vi "ConfigDevice.vi"(8 "error in (no error)":errorcluster, 11 "PacificPowerSource in":refnum<class "PacificPowerSource.lvclass">) -> (0 "error out":errorcluster, 3 "PacificPowerSource out":refnum<class "PacificPowerSource.lvclass">)   [LabVIEW 2018, in "AcPwrPlugins.lvlib" / "PacificPowerSource.lvclass"]
doc: "This VI configures the device based on the properties set in the preference dialog."
uses:
  PacificPowerSource.lvclass
  C:/Users/ico/Documents/Projects/NistPluggableModules/AcPwr/AcPwrPlugins/AcPwrBaseClass/AcPwrBase.lvclass
  AcPwrBaseClass/AcPwrBase.lvclass/AcPwrBase.ctl
  TypeDefs/ConfigDevicesModeSelection.ctl
  AcPwrBaseClass/Accessors/Read BaseConfig.vi
  <instrlib>/Pacific Power UPC Series/Pacific Power UPC Series.lvlib
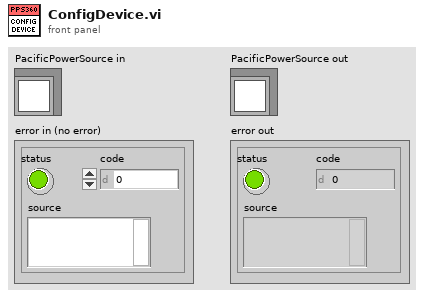
[diagram p1: front panel]
types:
  T1 = typedef "AcPwrPlugins.lvlib/PacificPowerSource.lvclass/ConfigDevicesModeSelection.ctl" = enum16{"Error", "ConfigureOutput", "VoltageLimit", "VoltageRange", "InitialVoltage", "FrequencyLimits", "FrequencyRange", "Impedance", "Waveform", "CustomWaveform", "Execute Program", "EnableOutput"}
  T2 = cluster{"Waveform 1":i32, "Waveform 2":i32, "Waveform 3":i32, "Voltage 1":dbl, "Voltage 2":dbl, "Voltage 3":dbl, "Phase 2":dbl, "Phase 3":dbl, "Frequency":dbl, "Current Limit":dbl, "# of Trans Events":i32, "Form":u16, "Coupling":u16, "XFMR Ratio":dbl, "Exec Angle":dbl}
  T3 = cluster{"Program Name":i32, "Waveform 1":i32, "Waveform 2":i32, "Waveform 3":i32, "Voltage 1":dbl, "Voltage 2":dbl, "Voltage 3":dbl, "Phase 2":dbl, "Phase 3":dbl, "Frequency":dbl, "Current Limit":dbl, "No. of Trans Events":i32, "Form":u16, "Coupling":u16, "XFMR Ratio":dbl, "Exec Angle":dbl}
  T4 = typedef "AcPwrPlugins.lvlib/AcPwrBase.lvclass/BaseConfig.ctl" = cluster{"Frequency":dbl, "FrequencyRange":dbl[], "Phases":T5[], "Name":string, "Chroma":T6, "NHRDC":T7, "PPS":T8, "PluginVariant":variant}
  T5 = typedef "AcPwrPlugins.lvlib/AcPwrBase.lvclass/Phase.ctl" = cluster{"Name":string, "Enabled":bool, "VoltageLevel":dbl, "Handle":string, "VoltageRange":dbl[], "Connected":bool, "CurrentLimit":dbl, "Waveform":string}
  T6 = typedef "AcPwrPlugins.lvlib/ChromaAcLoad.lvclass/DeviceProperties.ctl" = cluster{"Configuration Mode":enum16{"Constant Voltage (DC)", "Constant Power (DC)", "Constant Power (AC)", "Constant Current (DC)", "Constant Current (AC)", "Constant Resistance (DC)", "Constant Resistance (AC)", "Rectified Mode (DC)", "Inrush (AC)", "RLC CP (AC)", "RLC (AC)"}, "Phases":cluster{"Handle":string, "Name":string, "Phase Select":i32, "Instrument Options":string, "id query (T)":bool, "reset device (T)":bool, "Load Short Circuited":bool, "Line Synchronization":bool, "Load Current (A/Arms)":dbl, "Load Voltage (V/Vrms)":dbl, "Load Power (W)":dbl, "Load Resistance (Ohms)":dbl, "Load Current Peak Limit (A)":dbl, "Load Current Limit (A/Arms)":dbl, "Load Power Limit (W)":dbl, "Synch Frequency (Hz)":dbl, "Priority":enum16{"CF Only", "PF Only", "Both (CF)", "Both (PF)"}, "Crest Factor":dbl, "Power Factor":dbl, "Slew Rate":cluster{"Rise Slew Rate (A/ms)":i32, "Fall Slew Rate (A/ms)":i32}, "LC/RLC Mode":cluster{"Capacitance (uF)":i32, "Inductance (uH)":i32, "Series Resistance (Ohm)":dbl, "Parallel Resistance (Ohm)":dbl}, "Timing":cluster{"TimingOn":enum16{""}, "Hours":u32, "Minutes":u32, "Seconds":dbl, "CutoffVoltage":dbl}, "Connected":bool}[]}
  T7 = typedef "AcPwrPlugins.lvlib/NHRDCPower.lvclass/Device(s)Settings.ctl" = cluster{"Handle":string, "Name":string, "id query (Yes)":bool, "reset device (Yes)":bool, "Connected":bool, "Initial Battery Detect Voltage (0)":sgl, "SafetySettings":cluster{"SetWatchDog":bool, "Voltage (V)":sgl, "Current (A)":sgl, "Power (W)":sgl, "Voltage Delay (s)":sgl, "Current Delay (s)":sgl, "Power Delay (s)":sgl}, "Options String":string, "Aperture Time (s)":sgl, "operating state (Off)":i32, "OutputSettings":cluster{"Voltage (V)":sgl, "Current (A)":sgl, "Resistance (Ohms)":sgl, "Power (W)":sgl, "Enable Voltage":bool, "Enable Current":bool, "Enable Resistance":bool, "Enable Power":bool, "Delay After (s)":sgl, "Wait Value (V, A, W)":sgl, "Enable Wait":bool, "Wait on Value":i32}[], "SlewRate":cluster{"Set Voltage Rate V/S":dbl, "Set Current Rate A/S":dbl, "Set Resistance Rate R/S":dbl, "Set Power Rate W/S":dbl}}[]
  T8 = typedef "AcPwrPlugins.lvlib/PacificPowerSource.lvclass/DeviceSettings.ctl" = cluster{"Handle":string, "Connected":bool, "Clear Device (F)":bool, "btnIdQuery":bool, "btnReset":bool, "Program #":cluster{"Phase B (Degrees)":i32, "Waveform A (1: Sine)":i32, "Voltage Level (Va)":dbl, "Program Number (0)":i32, "Voltage Level (Vb) ":dbl, "Form (3: Three)":u16, "Coupling  (0: Direct)":u16, "Frequency (45Hz)":dbl, "Current Limit (40A)":dbl, "Phase C (Degrees)":i32, "Voltage Level (Vc)":dbl, "Waveform B (1: Sine)":i32, "Waveform C (1: Sine)":i32}[], "Impedance Parameters (off, 0.00)":cluster{"State":bool, "Impedance":dbl}, "Transient Execution (F)":bool, "OutputEnabled":bool, "Source Range":cluster{"Frequency Minimum (45 Hz)":dbl, "Frequency Maximum (1200 Hz)":dbl, "Voltage Maximum (V)":dbl, "Voltage Minimum (V)":dbl, "Range Control (0: Auto)":u16, "Initial Voltage (0V)":u16, "Frequency Range (600Hz)":u16}, "Port Type":enum16{"GPIB", "Serial"}}[]
  T9 = cluster{"Phase B (Degrees)":i32, "Waveform A (1: Sine)":i32, "Voltage Level (Va)":dbl, "Program Number (0)":i32, "Voltage Level (Vb) ":dbl, "Form (3: Three)":u16, "Coupling  (0: Direct)":u16, "Frequency (45Hz)":dbl, "Current Limit (40A)":dbl, "Phase C (Degrees)":i32, "Voltage Level (Vc)":dbl, "Waveform B (1: Sine)":i32, "Waveform C (1: Sine)":i32}[]
  T10 = cluster{"Phase B (Degrees)":i32, "Waveform A (1: Sine)":i32, "Voltage Level (Va)":dbl, "Program Number (0)":i32, "Voltage Level (Vb) ":dbl, "Form (3: Three)":u16, "Coupling  (0: Direct)":u16, "Frequency (45Hz)":dbl, "Current Limit (40A)":dbl, "Phase C (Degrees)":i32, "Voltage Level (Vc)":dbl, "Waveform B (1: Sine)":i32, "Waveform C (1: Sine)":i32}
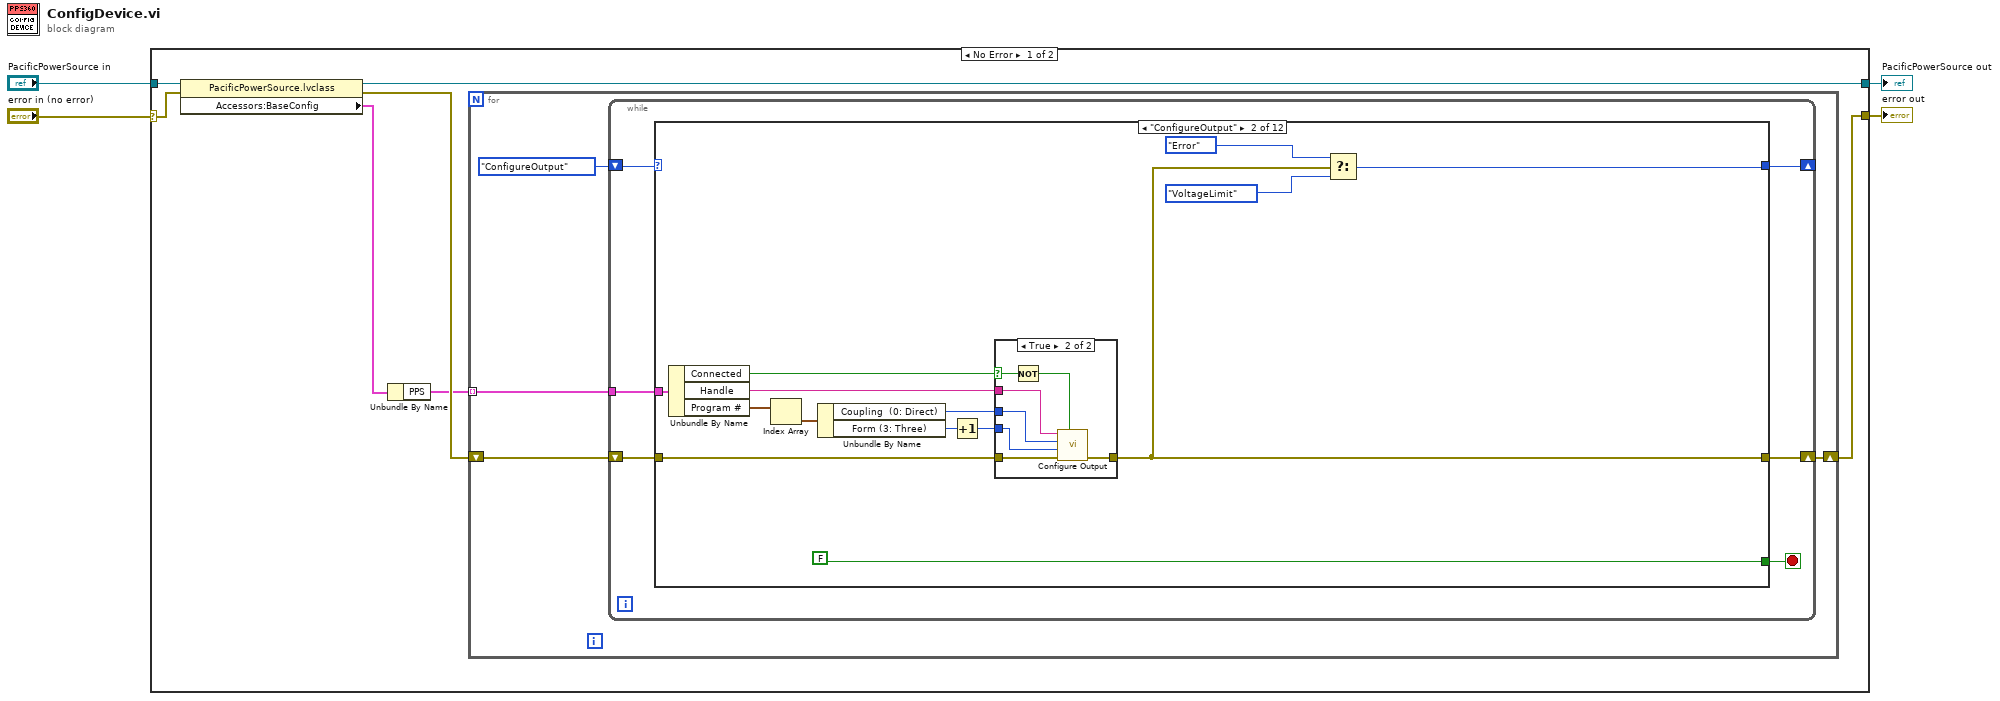
[diagram p0: block diagram]
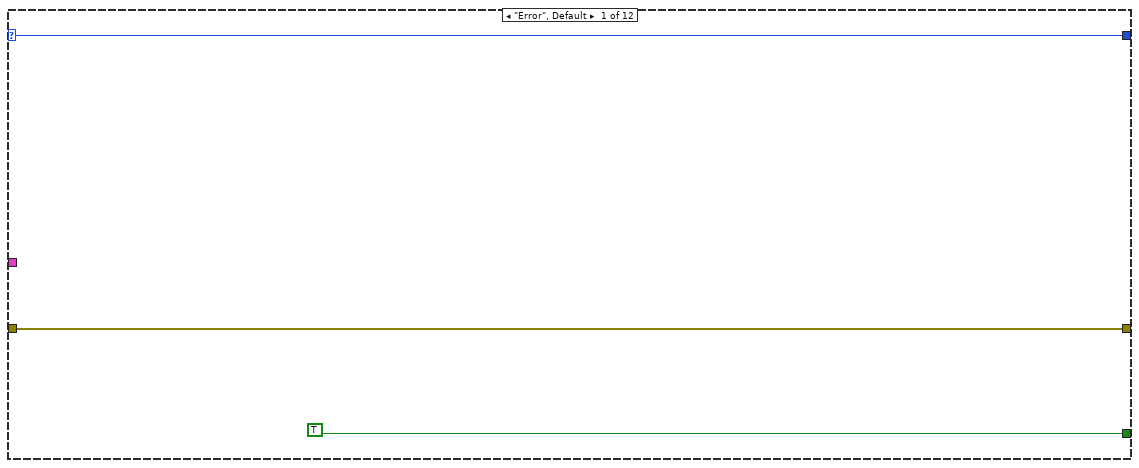
[diagram p2: hidden frame]
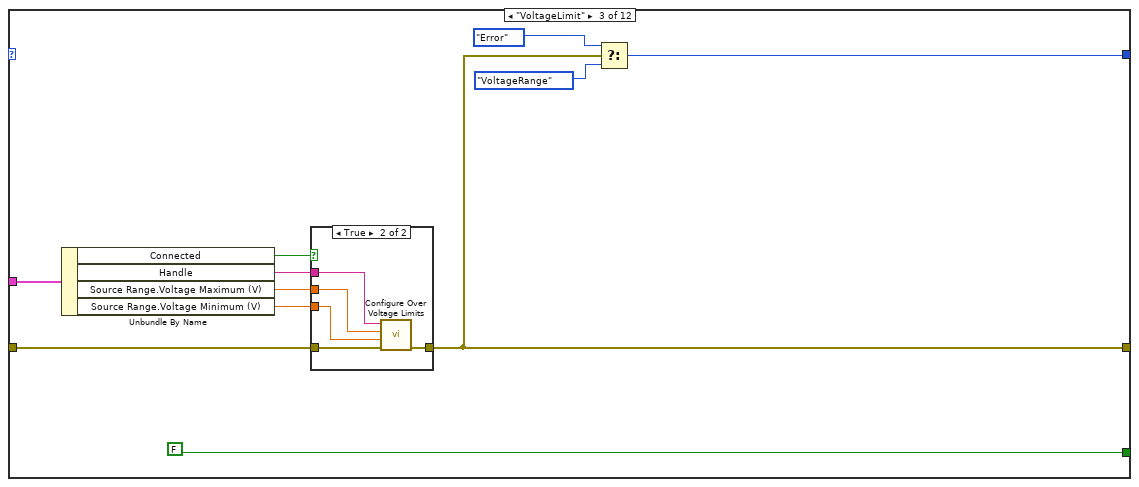
[diagram p4: hidden frame]
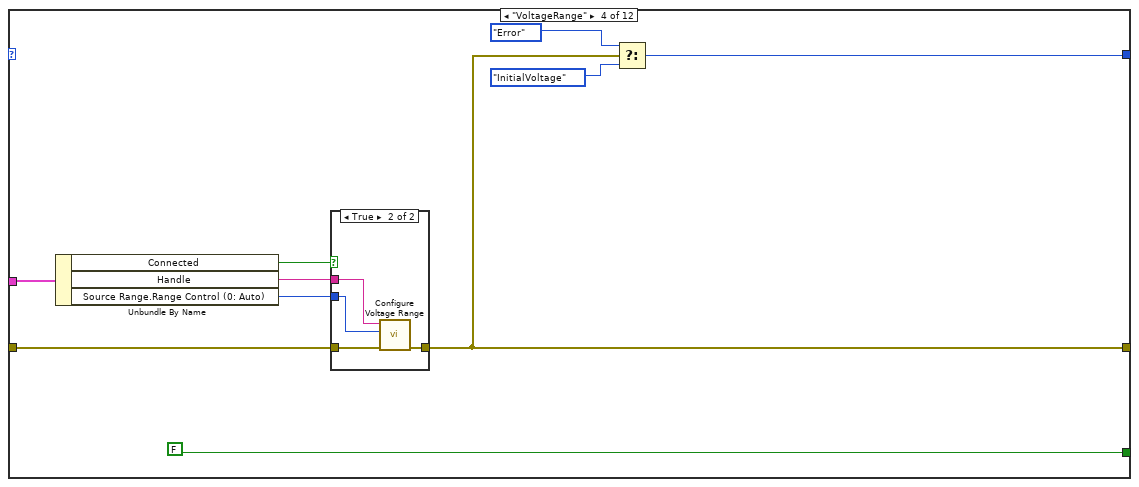
[diagram p6: hidden frame]
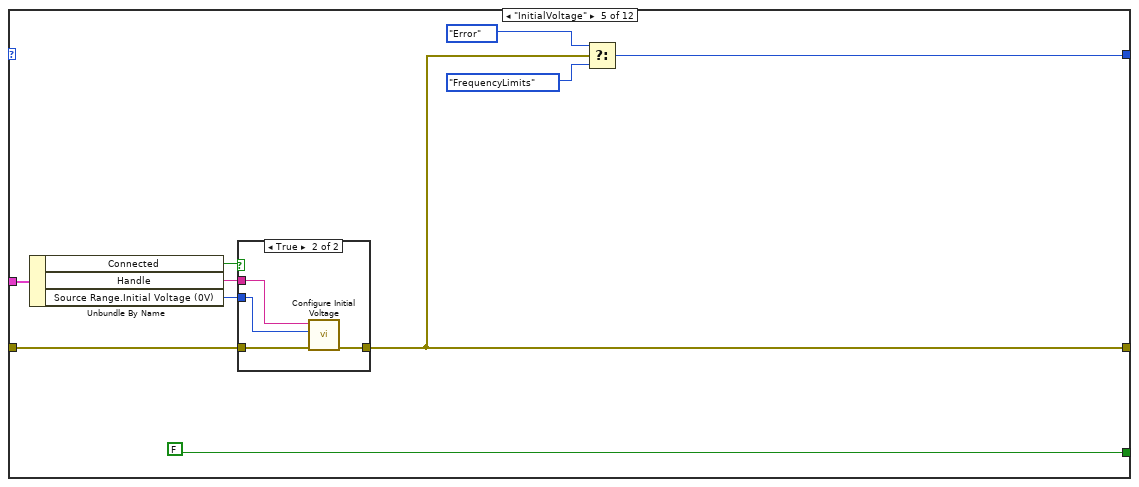
[diagram p8: hidden frame]
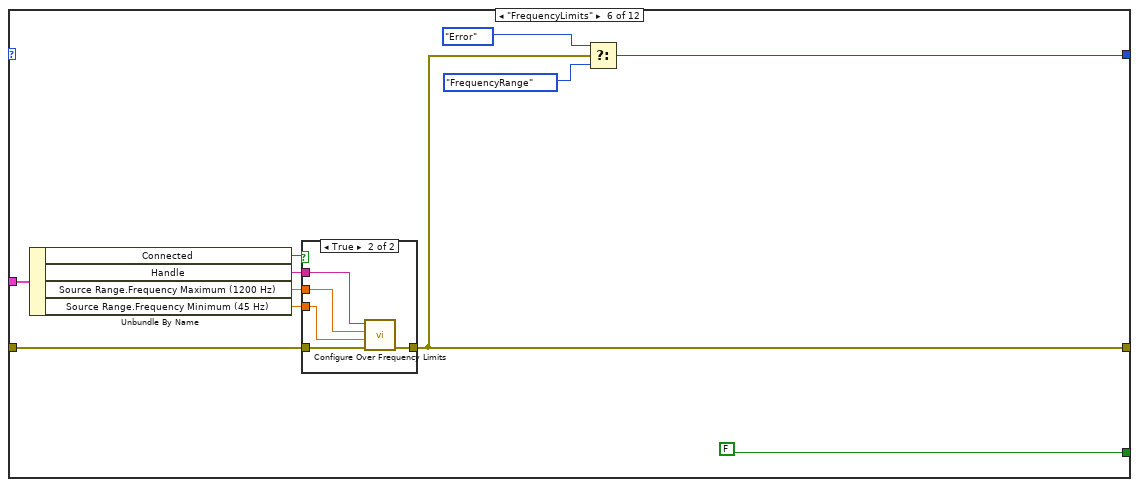
[diagram p10: hidden frame]
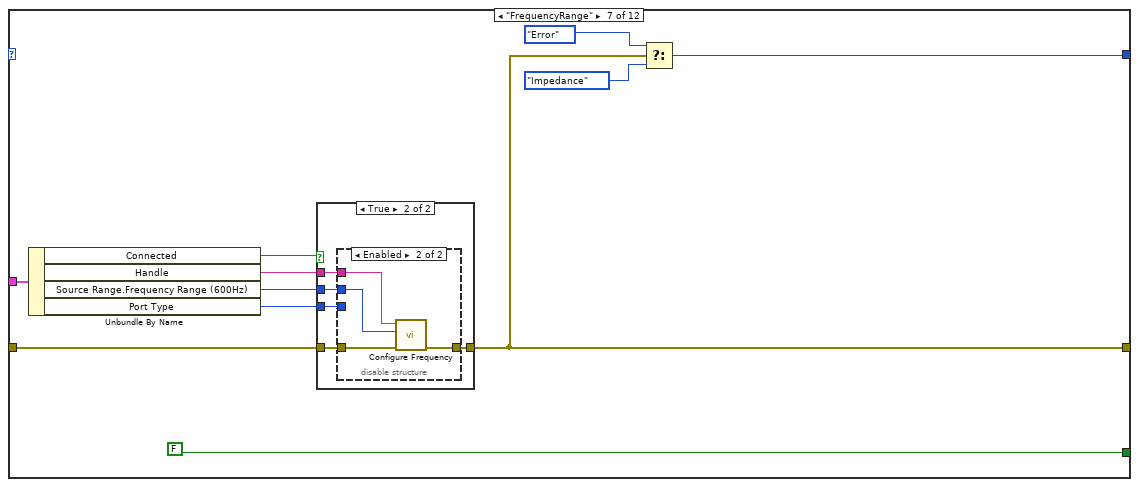
[diagram p12: hidden frame]
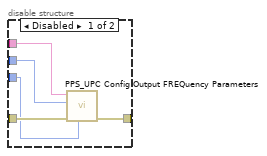
[diagram p14: hidden frame]
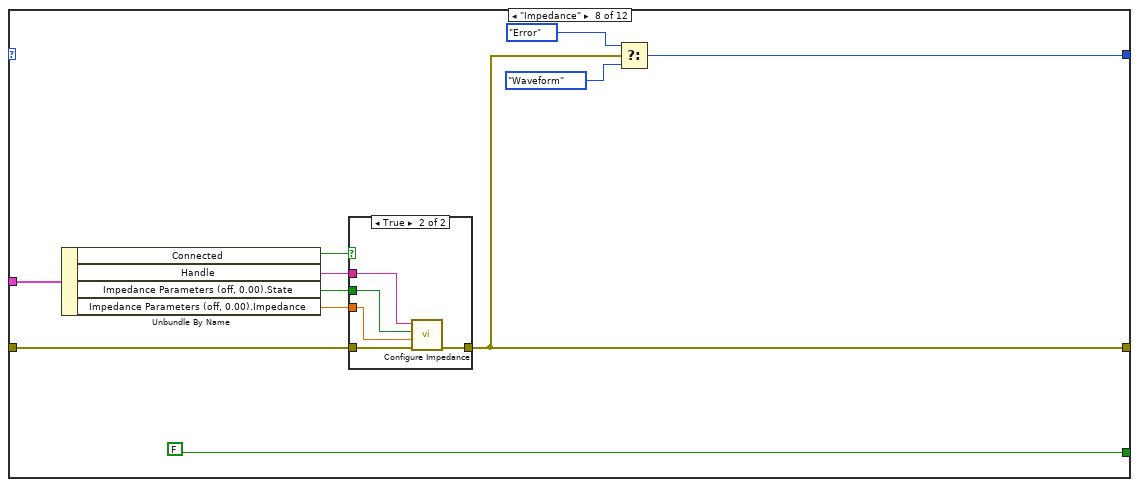
[diagram p15: hidden frame]
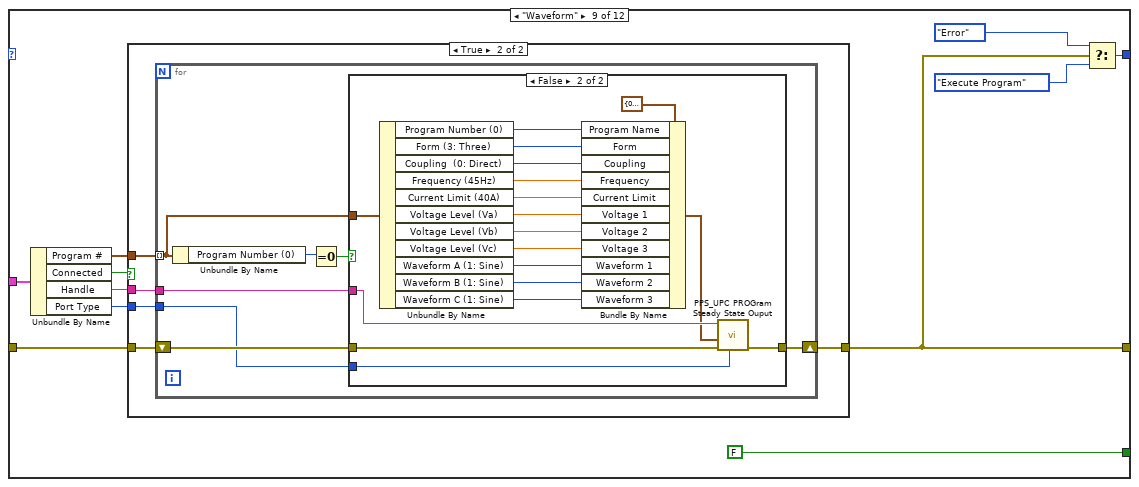
[diagram p17: hidden frame]
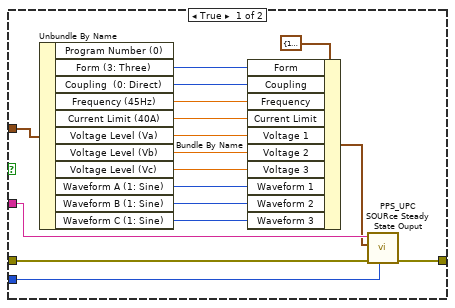
[diagram p19: hidden frame]
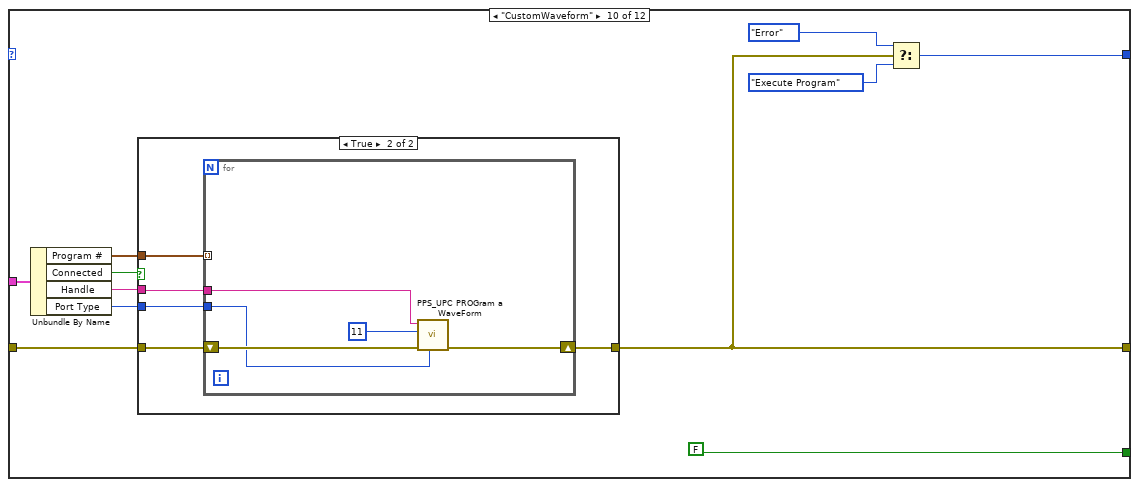
[diagram p20: hidden frame]
diagram:
  n1 = case shown="No Error" "error in (no error)" {
    selector: "error in (no error)" -> [w11 w278]
    tunnel: [w8 w278] -> w4
    tunnel: [w9 w277] -> w3
    tunnel: "PacificPowerSource in" -> [w10 w277]
    frame No Error {
      n2 = property class="PacificPowerSource.lvclass"(reference=w10, error in=w11) -> (reference out=w9:refnum<class "PacificPowerSource.lvclass">, error out=w7:errorcluster, "Accessors:BaseConfig"=w6:T4)
      n3 = Unbundle By Name(w6) -> ("PPS"=w5:T8)
      n4 = for {
        tunnel: w5 -> [w15] mode=indexing
        shift-right: [w13] -> w8
        shift-left: w7 -> [w14]
        n5 = while {
          tunnel: w15 -> [w21]
          shift-right: [w19] -> w13
          shift-left: w14 -> [w20]
          shift-right: [w16] -> _
          shift-left: ConfigDevicesModeSelection."ConfigureOutput" ("Enum") -> [w18]
          stop <- w17 stop-if-true
          n6 = case shown="\"ConfigureOutput\"" w18 {
            selector: w18 -> [w22 _ _ _ _ _ _ _ _ _ _ w259]
            tunnel: w21 -> [_ w32 w57 w73 w88 w104 w121 w140 w160 w219 w246 w264]
            tunnel: w20 -> [w24 w36 w54 w70 w84 w99 w117 w144 w162 w221 w247 w267]
            tunnel: [w24 w34 w52 w68 w82 w97 w115 w142 w155 w214 w244 w265] -> w19
            tunnel: [TRUE FALSE FALSE FALSE FALSE FALSE FALSE FALSE FALSE FALSE w235 TRUE] -> w17
            tunnel: [w22 w33 w51 w67 w81 w96 w114 w141 w156 w215 w242 w259] -> w16
            frame "Error", Default {
            }
            frame "ConfigureOutput" {
              n7 = Unbundle By Name(w32) -> ("Connected"=w38:bool, "Handle"=w37:string, "Program #"=w29:T9)
              n8 = Index Array(array=w29) -> (element=w28:T10)  [unwired: 1 in]
              n9 = Unbundle By Name(w28) -> ("Coupling  (0: Direct)"=w27:u16, "Form (3: Three)"=w26:u16)
              n10 = Increment(x=w26) -> (x+1=w25:u16)
              n11 = case shown="True" w38 {
                selector: w38 -> [_ w42]
                tunnel: w37 -> [_ w44]
                tunnel: w36 -> [w39 w45]
                tunnel: [w39 w46] -> w34
                tunnel: w27 -> [_ w43]
                tunnel: w25 -> [_ w40]
                frame False {
                }
                frame True {
                  n12 = Not(x=w42) -> (.not. x?=w41:bool)
                  n13 = call <instrlib>:"Configure Output.vi"("Enable Output (T: Enable)"=w41, "error in (no error)"=w45, "Form (3: Three)"=w40, "Coupling  (0: Direct)"=w43, "VISA resource name"=w44) -> ("error out"=w46:errorcluster)  [unwired: 5 in, 1 out]
                }
              }
              n14 = Select(t=ConfigDevicesModeSelection."Error" ("Enum"), s=w34, f=ConfigDevicesModeSelection."VoltageLimit" ("Enum")) -> (s? t:f=w33:T1)
            }
            frame "VoltageLimit" {
              n15 = Unbundle By Name(w57) -> ("Connected"=w50:bool, "Handle"=w56:string, "Source Range.Voltage Maximum (V)"=w55:dbl, "Source Range.Voltage Minimum (V)"=w49:dbl)
              n16 = case shown="True" w50 {
                tunnel: w56 -> [_ w61]
                tunnel: w55 -> [_ w60]
                tunnel: w54 -> [w58 w63]
                tunnel: [w58 w62] -> w52
                tunnel: w49 -> [_ w59]
                frame False {
                }
                frame True {
                  n17 = call <instrlib>:"Configure Over Voltage Limits.vi"("error in (no error)"=w63, "Low Limit (0.0 V)"=w59, "High Limit (600.0 V)"=w60, "VISA resource name"=w61) -> ("error out"=w62:errorcluster)  [unwired: 6 in, 1 out]
                }
              }
              n18 = Select(t=ConfigDevicesModeSelection."Error" ("Enum"), s=w52, f=ConfigDevicesModeSelection."VoltageRange" ("Enum")) -> (s? t:f=w51:T1)
            }
            frame "VoltageRange" {
              n19 = Unbundle By Name(w73) -> ("Connected"=w66:bool, "Handle"=w72:string, "Source Range.Range Control (0: Auto)"=w71:u16)
              n20 = case shown="True" w66 {
                tunnel: w72 -> [_ w76]
                tunnel: w71 -> [_ w75]
                tunnel: w70 -> [w74 w78]
                tunnel: [w74 w77] -> w68
                frame False {
                }
                frame True {
                  n21 = call <instrlib>:"Configure Voltage Range.vi"("error in (no error)"=w78, "Range Control (0: Auto)"=w75, "VISA resource name"=w76) -> ("error out"=w77:errorcluster)  [unwired: 7 in, 1 out]
                }
              }
              n22 = Select(t=ConfigDevicesModeSelection."Error" ("Enum"), s=w68, f=ConfigDevicesModeSelection."InitialVoltage" ("Enum")) -> (s? t:f=w67:T1)
            }
            frame "InitialVoltage" {
              n23 = Unbundle By Name(w88) -> ("Connected"=w87:bool, "Handle"=w86:string, "Source Range.Initial Voltage (0V)"=w85:u16)
              n24 = case shown="True" w87 {
                tunnel: w86 -> [_ w91]
                tunnel: w85 -> [_ w90]
                tunnel: w84 -> [w89 w92]
                tunnel: [w89 w93] -> w82
                frame False {
                }
                frame True {
                  n25 = call <instrlib>:"Configure Initial Voltage.vi"("error in (no error)"=w92, "Initial Voltage (0: 0 V)"=w90, "VISA resource name"=w91) -> ("error out"=w93:errorcluster)  [unwired: 7 in, 1 out]
                }
              }
              n26 = Select(t=ConfigDevicesModeSelection."Error" ("Enum"), s=w82, f=ConfigDevicesModeSelection."FrequencyLimits" ("Enum")) -> (s? t:f=w81:T1)
            }
            frame "FrequencyLimits" {
              n27 = Unbundle By Name(w104) -> ("Connected"=w103:bool, "Handle"=w102:string, "Source Range.Frequency Maximum (1200 Hz)"=w101:dbl, "Source Range.Frequency Minimum (45 Hz)"=w100:dbl)
              n28 = case shown="True" w103 {
                tunnel: w102 -> [_ w108]
                tunnel: w101 -> [_ w107]
                tunnel: w100 -> [_ w106]
                tunnel: w99 -> [w105 w109]
                tunnel: [w105 w110] -> w97
                frame False {
                }
                frame True {
                  n29 = call <instrlib>:"Configure Over Frequency Limits.vi"("error in (no error)"=w109, "Low Limit (45.0 Hz)"=w106, "High Limit (1200.0 Hz)"=w107, "VISA resource name"=w108) -> ("error out"=w110:errorcluster)  [unwired: 6 in, 1 out]
                }
              }
              n30 = Select(t=ConfigDevicesModeSelection."Error" ("Enum"), s=w97, f=ConfigDevicesModeSelection."FrequencyRange" ("Enum")) -> (s? t:f=w96:T1)
            }
            frame "FrequencyRange" {
              n31 = Unbundle By Name(w121) -> ("Connected"=w120:bool, "Handle"=w119:string, "Source Range.Frequency Range (600Hz)"=w118:u16, "Port Type"=w111:enum16{"GPIB", "Serial"})
              n32 = case shown="True" w120 {
                tunnel: w119 -> [_ w123]
                tunnel: w118 -> [_ w125]
                tunnel: w117 -> [w122 w126]
                tunnel: [w122 w127] -> w115
                tunnel: w111 -> [_ w124]
                frame False {
                }
                frame True {
                  n33 = disable-structure shown="Enabled" {
                    disable-tunnel: [w132 w135] -> w127
                    disable-tunnel: w126 -> [w131 w136]
                    disable-tunnel: w125 -> [w130 w133]
                    disable-tunnel: w124 -> [w129 _]
                    disable-tunnel: w123 -> [w128 w134]
                    frame Disabled {
                      n34 = call <instrlib>:"PPS_UPC Config Output FREQuency Parameters.vi"("Port Type"=w129, "error in (no error)"=w131, "Frequency Span (600)"=w130, "VISA session"=w128) -> ("error out"=w132:errorcluster)  [unwired: 6 in, 1 out]
                    }
                    frame Enabled {
                      n35 = call <instrlib>:"Configure Frequency.vi"("error in (no error)"=w136, "Frequency Range (600 Hz)"=w133, "VISA resource name"=w134) -> ("error out"=w135:errorcluster)  [unwired: 7 in, 1 out]
                    }
                  }
                }
              }
              n36 = Select(t=ConfigDevicesModeSelection."Error" ("Enum"), s=w115, f=ConfigDevicesModeSelection."Impedance" ("Enum")) -> (s? t:f=w114:T1)
            }
            frame "Impedance" {
              n37 = Unbundle By Name(w140) -> ("Connected"=w147:bool, "Handle"=w146:string, "Impedance Parameters (off, 0.00).State"=w145:bool, "Impedance Parameters (off, 0.00).Impedance"=w139:dbl)
              n38 = case shown="True" w147 {
                tunnel: w146 -> [_ w151]
                tunnel: w145 -> [_ w150]
                tunnel: w144 -> [w148 w152]
                tunnel: [w148 w153] -> w142
                tunnel: w139 -> [_ w149]
                frame False {
                }
                frame True {
                  n39 = call <instrlib>:"Configure Impedance.vi"("error in (no error)"=w152, "Output Impedance (0.0 Ohm)"=w149, "Enable Impedance (T: Enable)"=w150, "VISA resource name"=w151) -> ("error out"=w153:errorcluster)  [unwired: 6 in, 1 out]
                }
              }
              n40 = Select(t=ConfigDevicesModeSelection."Error" ("Enum"), s=w142, f=ConfigDevicesModeSelection."Waveform" ("Enum")) -> (s? t:f=w141:T1)
            }
            frame "Waveform" {
              n41 = Unbundle By Name(w160) -> ("Program #"=w159:T9, "Connected"=w164:bool, "Handle"=w163:string, "Port Type"=w154:enum16{"GPIB", "Serial"})
              n42 = case shown="True" w164 {
                tunnel: w163 -> [_ w168]
                tunnel: w162 -> [w165 w169]
                tunnel: [w165 w170] -> w155
                tunnel: w159 -> [_ w167]
                tunnel: w154 -> [_ w166]
                frame False {
                }
                frame True {
                  n43 = for {
                    shift-right: [w176] -> w170
                    shift-left: w169 -> [w177]
                    tunnel: w168 -> [w173]
                    tunnel: w167 -> [w172] mode=indexing
                    tunnel: w166 -> [w171]
                    n44 = Unbundle By Name(w172) -> ("Program Number (0)"=w175:i32)
                    n45 = Equal To 0?(x=w175) -> (x = 0?=w174:bool)
                    n46 = case shown="False" w174 {
                      tunnel: w177 -> [w194 w212]
                      tunnel: [w193 w201] -> w176
                      tunnel: w171 -> [w192 w200]
                      tunnel: w173 -> [w191 w199]
                      tunnel: w172 -> [w189 w211]
                      frame True {
                        n47 = Unbundle By Name(w189) -> ("Form (3: Three)"=w179:u16, "Coupling  (0: Direct)"=w180:u16, "Frequency (45Hz)"=w184:dbl, "Current Limit (40A)"=w185:dbl, "Voltage Level (Va)"=w188:dbl, "Voltage Level (Vb)"=w187:dbl, "Voltage Level (Vc)"=w186:dbl, "Waveform A (1: Sine)"=w183:i32, "Waveform B (1: Sine)"=w182:i32, "Waveform C (1: Sine)"=w181:i32)  [unwired: 1 out]
                        n48 = Bundle By Name(cluster=T2 {"Waveform 1"=1, "Waveform 2"=1, "Waveform 3"=1, "Voltage 1"=100.0, "Voltage 2"=100.0, "Voltage 3"=100.0, "Phase 2"=120.0, "Phase 3"=240.0, "Frequency"=100.0, "Current Limit"=10.0, "# of Trans Events"=0, "Form"=0, "Coupling"=0, "XFMR Ratio"=0.0, "Exec Angle"=0.0} ("Steady State Output Parameters 2"), "Form"=w179, "Coupling"=w180, "Frequency"=w184, "Current Limit"=w185, "Voltage 1"=w188, "Voltage 2"=w187, "Voltage 3"=w186, "Waveform 1"=w183, "Waveform 2"=w182, "Waveform 3"=w181) -> (w190:T2)
                        n49 = call <instrlib>:"PPS_UPC SOURce Steady State Ouput.vi"("Port Type"=w192, "error in (no error)"=w194, "Steady State\nOutput Parameters"=w190, "VISA session"=w191) -> ("error out"=w193:errorcluster)  [unwired: 6 in, 1 out]
                      }
                      frame False {
                        n50 = Unbundle By Name(w211) -> ("Program Number (0)"=w197:i32, "Form (3: Three)"=w198:u16, "Coupling  (0: Direct)"=w202:u16, "Frequency (45Hz)"=w206:dbl, "Current Limit (40A)"=w207:dbl, "Voltage Level (Va)"=w210:dbl, "Voltage Level (Vb)"=w209:dbl, "Voltage Level (Vc)"=w208:dbl, "Waveform A (1: Sine)"=w205:i32, "Waveform B (1: Sine)"=w204:i32, "Waveform C (1: Sine)"=w203:i32)
                        n51 = Bundle By Name(cluster=T3 {"Program Name"=0, "Waveform 1"=0, "Waveform 2"=0, "Waveform 3"=0, "Voltage 1"=0.0, "Voltage 2"=0.0, "Voltage 3"=0.0, "Phase 2"=0.0, "Phase 3"=0.0, "Frequency"=0.0, "Current Limit"=0.0, "No. of Trans Events"=0, "Form"=0, "Coupling"=0, "XFMR Ratio"=0.0, "Exec Angle"=0.0} ("Program Steady State Parameters"), "Program Name"=w197, "Form"=w198, "Coupling"=w202, "Frequency"=w206, "Current Limit"=w207, "Voltage 1"=w210, "Voltage 2"=w209, "Voltage 3"=w208, "Waveform 1"=w205, "Waveform 2"=w204, "Waveform 3"=w203) -> (w196:T3)
                        n52 = call <instrlib>:"PPS_UPC PROGram Steady State Ouput.vi"("Port Type"=w200, "error in (no error)"=w212, "Program Steady State Parameters"=w196, "VISA session"=w199) -> ("error out"=w201:errorcluster)  [unwired: 6 in, 1 out]
                      }
                    }
                  }
                }
              }
              n53 = Select(t=ConfigDevicesModeSelection."Error" ("Enum"), s=w155, f=ConfigDevicesModeSelection."Execute Program" ("Enum")) -> (s? t:f=w156:T1)
            }
            frame "CustomWaveform" {
              n54 = Unbundle By Name(w219) -> ("Program #"=w218:T9, "Connected"=w223:bool, "Handle"=w222:string, "Port Type"=w213:enum16{"GPIB", "Serial"})
              n55 = case shown="True" w223 {
                tunnel: w222 -> [_ w227]
                tunnel: w221 -> [w224 w228]
                tunnel: [w224 w229] -> w214
                tunnel: w218 -> [_ w226]
                tunnel: w213 -> [_ w225]
                frame False {
                }
                frame True {
                  n56 = for {
                    shift-right: [w232] -> w229
                    shift-left: w228 -> [w234]
                    tunnel: w227 -> [w233]
                    tunnel: w226 -> [_] mode=indexing
                    tunnel: w225 -> [w230]
                    n57 = call <instrlib>:"PPS_UPC PROGram a WaveForm.vi"("Port Type"=w230, "error in (no error)"=w234, "Waveform Name"=11, "VISA session"=w233) -> ("error out"=w232:errorcluster)  [unwired: 6 in, 1 out]
                  }
                }
              }
              n58 = Select(t=ConfigDevicesModeSelection."Error" ("Enum"), s=w214, f=ConfigDevicesModeSelection."Execute Program" ("Enum")) -> (s? t:f=w215:T1)
            }
            frame "Execute Program" {
              n59 = Unbundle By Name(w246) -> ("OutputEnabled"=w237:bool, "Connected"=w249:bool, "Handle"=w248:string, "Program #"=w241:T9, "Port Type"=w238:enum16{"GPIB", "Serial"})
              n60 = Index Array(array=w241) -> (element=w240:T10)  [unwired: 1 in]
              n61 = Unbundle By Name(w240) -> ("Program Number (0)"=w239:i32)
              n62 = case shown="True" w249 {
                tunnel: w248 -> [_ w254]
                tunnel: w247 -> [w251 w257]
                tunnel: [w251 w256] -> w244
                tunnel: w239 -> [_ w255]
                tunnel: w238 -> [_ w253]
                tunnel: w237 -> [w250 w252]
                tunnel: [w250 w252] -> w236
                frame False {
                }
                frame True {
                  n63 = call <instrlib>:"PPS_UPC EXECute PROGram.vi"("Port Type"=w253, "error in (no error)"=w257, "Program Name (1)"=w255, "VISA session"=w254) -> ("error out"=w256:errorcluster)  [unwired: 6 in, 1 out]
                }
              }
              n64 = Not(x=w236) -> (.not. x?=w235:bool)
              n65 = Select(t=ConfigDevicesModeSelection."Error" ("Enum"), s=w244, f=ConfigDevicesModeSelection."EnableOutput" ("Enum")) -> (s? t:f=w242:T1)
            }
            frame "EnableOutput" {
              n66 = Unbundle By Name(w264) -> ("Connected"=w269:bool, "Handle"=w268:string, "Program #"=w263:T9)
              n67 = Index Array(array=w263) -> (element=w262:T10)  [unwired: 1 in]
              n68 = Unbundle By Name(w262) -> ("Coupling  (0: Direct)"=w261:u16, "Form (3: Three)"=w260:u16)
              n69 = Increment(x=w260) -> (x+1=w258:u16)
              n70 = case shown="True" w269 {
                tunnel: w268 -> [_ w274]
                tunnel: w267 -> [w270 w275]
                tunnel: [w270 w276] -> w265
                tunnel: w261 -> [_ w272]
                tunnel: w258 -> [_ w271]
                frame False {
                }
                frame True {
                  n71 = call <instrlib>:"Configure Output.vi"("Enable Output (T: Enable)"=TRUE, "error in (no error)"=w275, "Form (3: Three)"=w271, "Coupling  (0: Direct)"=w272, "VISA resource name"=w274) -> ("error out"=w276:errorcluster)  [unwired: 5 in, 1 out]
                }
              }
            }
          }
        }
      }
    }
    frame Error {
    }
  }
  "error out" <- w4
  "PacificPowerSource out" <- w3
